vi "Channel Config Page.vi"(8 "error in (no error)":errorcluster, 11 "Node Ptr":T1 format="%.0x") -> (0 "error out":errorcluster)   [LabVIEW 2016, in "UDP-Custom-Device System Explorer.lvlib"]
uses:
  UDP-Custom-Device System Explorer.lvlib
  <vilib>/NI Veristand/Custom Device API/Custom Device Item Ref.ctl
  <vilib>/NI VeriStand/Custom Device API/Custom Device API.lvlib
  <vilib>/NI VeriStand/Custom Device Tools/Custom Device Utility Library/Custom Device Utility Library.lvlib
panel:
  out "Imported Channel Configuration":i32[](listbox) caption="Channels"
  in  "Channel Configuration File":path
  in  "Description":string
  out "Name":string
  in  "SHDocVw.IWebBrowser":refnum<k7>(container)
  in  "General Header":cluster{"Section Name":string}={"Section Name"="Channel Configuration"}
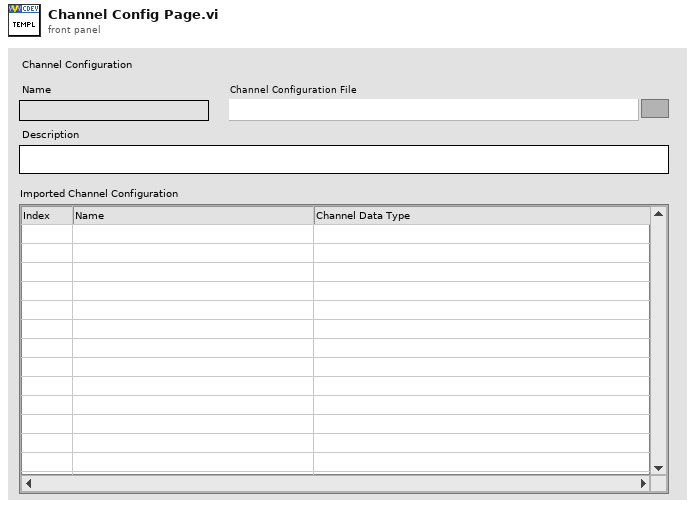
[diagram p1: front panel]
types:
  T1 = typedef "Custom Device API.lvlib/Custom Device Item Ref.ctl" = u64
  T2 = typedef "Custom Device API.lvlib/Custom Device Commands.ctl" = enum16{"Default", "Item renamed", "Shutdown", "Dynamic button pressed"}
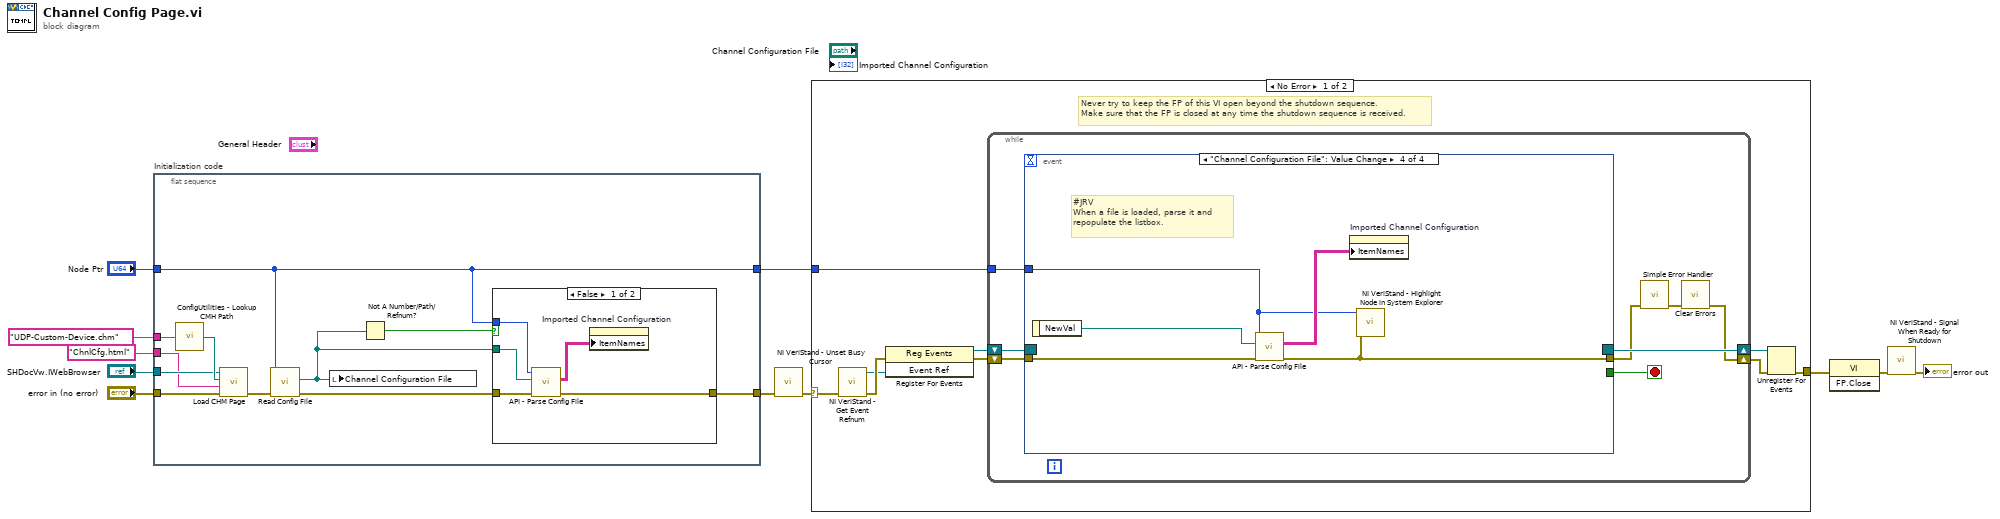
[diagram p0: block diagram]
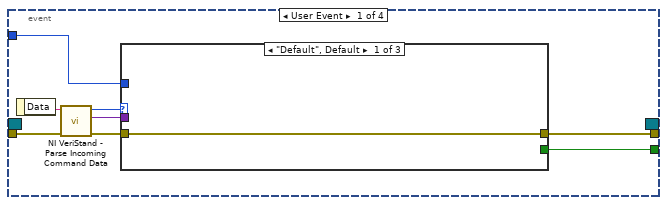
[diagram p3: hidden frame]
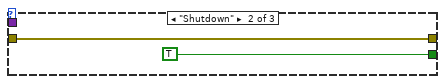
[diagram p4: hidden frame]
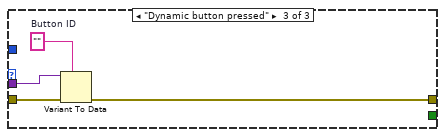
[diagram p5: hidden frame]
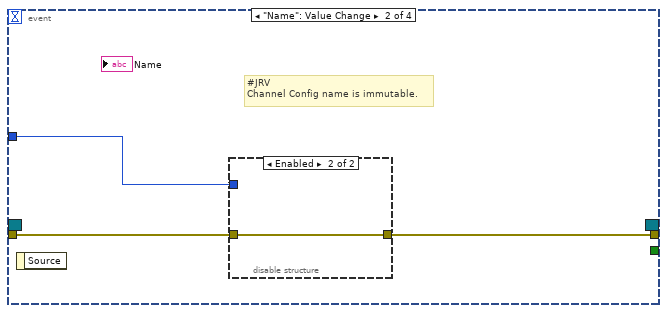
[diagram p6: hidden frame]
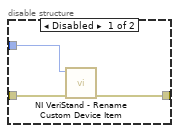
[diagram p7: hidden frame]
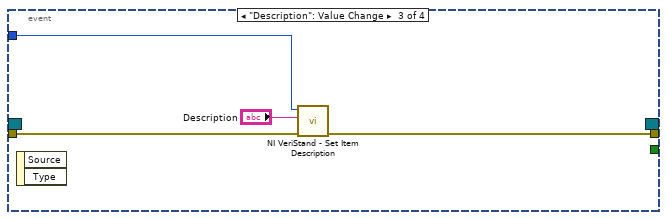
[diagram p8: hidden frame]
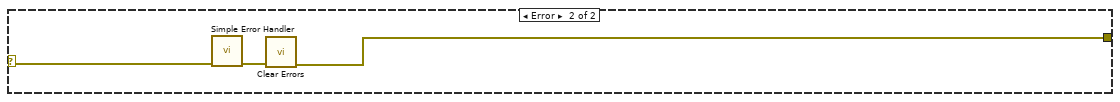
[diagram p9: hidden frame]
diagram:
  n1 = flat-sequence "Initialization code" {
    tunnel: "error in (no error)" -> [w21]
    tunnel: "Node Ptr" -> [w12]
    tunnel: [w16] -> w7
    tunnel: [w12] -> w4
    tunnel: "SHDocVw.IWebBrowser" -> [w20]
    tunnel: "ChnlCfg.html" ("CD_CHM_Section") -> [w18]
    tunnel: "UDP-Custom-Device.chm" ("CD_CHM_FileName") -> [w19]
    frame #0 {
      n2 = call "ConfigUtilities - Lookup CMH Path.vi"("Main CMH File"=w19) -> ("Compiled CMH Path"=w22:path)
      n3 = call <vilib>:"Load CHM Page.vi"("error in (no error)"=w21, "HTML File"=w18, "Compiled CHM Path"=w22, "Web Browser Reference"=w20) -> ("error out"=w17:errorcluster)  [unwired: 7 in]
      n4 = call "Read Config File.vi"("error in (no error)"=w17, "Node Ptr"=w12) -> ("error out"=w15:errorcluster, "Config File"=w13:path)  [unwired: 7 in, 1 out]
      n5 = local write "Channel Configuration File"(w13) -> ()
      n6 = Not A Number/Path/Refnum?(number/path/refnum=w13) -> (NaN/Path/Refnum?=w14:bool)
      n7 = case shown="False" w14 {
        tunnel: [w24 w28] -> w16
        tunnel: w15 -> [w25 w28]
        tunnel: w13 -> [w27 _]
        tunnel: w12 -> [w26 _]
        frame False {
          n8 = call "API - Parse Config File.vi"("error in (no error)"=w25, "Config Path"=w27, "Node Ptr"=w26) -> ("error out"=w24:errorcluster, "Channel Configuration"=w23:string[][])  [unwired: 6 in, 1 out]
          n9 = property on="Imported Channel Configuration" class="MCListbox (strict)"("ItemNames"=w23) -> ()  [unwired: 2 in, 2 out]
        }
        frame True {
        }
      }
    }
  }
  n10 = call <vilib>:"NI VeriStand - Unset Busy Cursor.vi"("error in (no error)"=w7) -> ("error out"=w6:errorcluster)  [unwired: 10 out]
  n11 = case shown="No Error" w6 {
    selector: w6 -> [w29 w79]
    tunnel: [w34 w77] -> w11
    tunnel: w4 -> [w30 _]
    frame No Error {
      # "Never try to keep the FP of this VI open beyond the shutdown sequence.\nMake sure that the FP is closed at any time the shutdown sequence is received."
      n12 = call <vilib>:"NI VeriStand - Get Event Refnum.vi"("error in (no error)"=w29) -> ("error out"=w37:errorcluster, "Event Ref"=w33:refnum<user-event>)  [unwired: 9 out]
      n13 = register-events(error in=w37, w33) -> (reference out=w31:refnum<event-registration>, error out=w32:errorcluster)  [unwired: 1 in]
      n14 = while {
        tunnel: w30 -> [w41]
        shift-right: [w38] -> w35
        shift-left: w32 -> [w44]
        shift-right: [w45] -> w36
        shift-left: w31 -> [w43]
        stop <- w42 stop-if-true
        n15 = event shown="[3] \"Channel Configuration File\": Value Change" {
          selector: w43 -> [_ _ _ _]
          dyn-events: [_ _ _ _] -> w45
          timeout: _ -> [_ _ _ _]
          tunnel: w44 -> [w53 w63 w71 w76]
          tunnel: [w49 _ _ _] -> w42
          tunnel: [w48 w61 w68 w72] -> w40
          tunnel: w41 -> [w47 w62 w70 w73]
          event User Event {
            n16 = event-data() -> ("Data"=w52:string)  [unwired: 1 out]
            n17 = call <vilib>:"NI VeriStand - Parse Incoming Command Data.vi"("error in (no error)"=w53, "Incoming data"=w52) -> ("error out"=w51:errorcluster, "Outgoing data"=w46:variant, "Action"=w50:T2)  [unwired: 7 out]
            n18 = case shown="\"Default\", Default" w50 {
              tunnel: w51 -> [w54 w55 w60]
              tunnel: [_ TRUE _] -> w49
              tunnel: [w54 w55 w57] -> w48
              tunnel: w47 -> [_ _ _]
              tunnel: w46 -> [_ _ w59]
              frame "Default", Default {
              }
              frame "Shutdown" {
              }
              frame "Dynamic button pressed" {
                w58 = ""  # Button ID
                n19 = Variant To Data(error in=w60, type=w58, Variant=w59) -> (error out=w57:errorcluster)  [unwired: 1 out]
              }
            }
          }
          event "Name": Value Change {
            # "#JRV\nChannel Config name is immutable."
            n20 = event-data() -> ()  [unwired: 2 out]
            n21 = disable-structure shown="Enabled" {
              disable-tunnel: w63 -> [w66 w67]
              disable-tunnel: w62 -> [w65 _]
              disable-tunnel: [w64 w67] -> w61
              frame Disabled {
                n22 = call <vilib>:"NI VeriStand - Rename Custom Device Item.vi"("error in (no error)"=w66, "Item Ref in"=w65) -> ("error out"=w64:errorcluster)  [unwired: 7 in, 2 out]
              }
              frame Enabled {
              }
            }
          }
          event "Description": Value Change {
            n23 = event-data() -> ()  [unwired: 3 out]
            n24 = call <vilib>:"NI VeriStand - Set Item Description.vi"("error in (no error)"=w71, "Description"="Description", "Item Ref in"=w70) -> ("error out"=w68:errorcluster)  [unwired: 6 in, 2 out]
          }
          event "Channel Configuration File": Value Change {
            # "#JRV\nWhen a file is loaded, parse it and\nrepopulate the listbox."
            n25 = event-data() -> ("NewVal"=w75:path)  [unwired: 1 out]
            n26 = call "API - Parse Config File.vi"("error in (no error)"=w76, "Config Path"=w75, "Node Ptr"=w73) -> ("error out"=w72:errorcluster, "Channel Configuration"=w74:string[][])  [unwired: 6 in, 1 out]
            n27 = property on="Imported Channel Configuration" class="MCListbox (strict)"("ItemNames"=w74) -> ()  [unwired: 2 in, 2 out]
            n28 = call <vilib>:"NI VeriStand - Highlight Node in System Explorer.vi"("error in (no error)"=w72, "Item Ref in"=w73) -> ()  [unwired: 8 in, 2 out]
          }
        }
        n29 = call <vilib>:"Simple Error Handler.vi"("error in (no error)"=w40) -> ("error out"=w39:errorcluster)  [unwired: 1 in, 7 out]
        n30 = call <vilib>:"Clear Errors.vi"("error in (no error)"=w39) -> ("error out"=w38:errorcluster)  [unwired: 1 in, 5 out]
      }
      n31 = Unregister For Events(event registration refnum=w36, error in=w35) -> (error out=w34:errorcluster)
    }
    frame Error {
      n32 = call <vilib>:"Simple Error Handler.vi"("error in (no error)"=w79) -> ("error out"=w78:errorcluster)  [unwired: 1 in, 7 out]
      n33 = call <vilib>:"Clear Errors.vi"("error in (no error)"=w78) -> ("error out"=w77:errorcluster)  [unwired: 1 in, 5 out]
    }
  }
  n34 = invoke class="VI" method="FP.Close"(error in=w11) -> (error out=w10:errorcluster)  [unwired: 2 in, 2 out]
  n35 = call <vilib>:"NI VeriStand - Signal When Ready for Shutdown.vi"("error in (no error)"=w10) -> ("error out"=→"error out":errorcluster)  [unwired: 10 out]
